vi "SENS_CORR_COLL_GUID_CONN_CAT_ARY.vi"(0 "VNA":refnum<visa-resource-name>, 5 "error in":errorcluster, 7 "Channel":i32) -> (14 "VNA Out":refnum<visa-resource-name>, 16 "ConAry":string[](array[string]), 19 "error out":errorcluster)   [LabVIEW 2018, in "PNA-X.lvlib"]
uses:
  PNA-X.lvlib
panel:
  out "read buffer":string
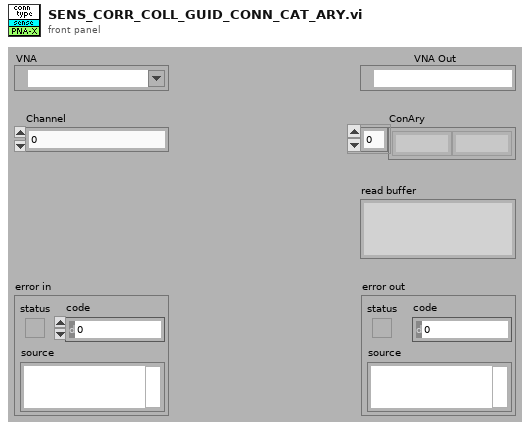
[diagram p1: front panel]
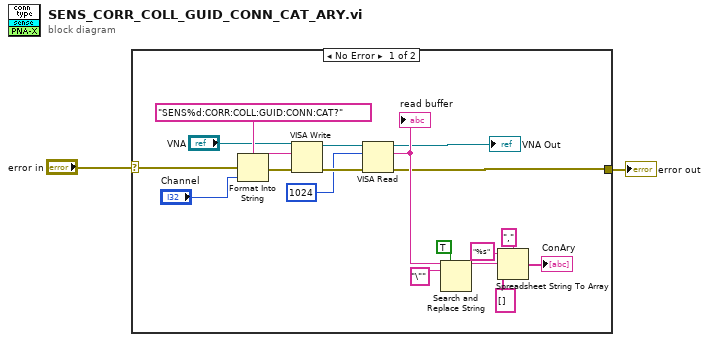
[diagram p0: block diagram]
diagram:
  n1 = case shown="No Error" "error in" {
    selector: "error in" -> [w6 w22]
    tunnel: [w3 w22] -> w1
    frame No Error {
      n2 = Format Into String(format string="SENS%d:CORR:COLL:GUID:CONN:CAT?", error in=w6, "Channel") -> (resulting string=w18:string, error out=w19:errorcluster)  [unwired: 1 in]
      n3 = VISA Write(VISA resource name="VNA", write buffer=w18, error in (no error)=w19) -> (VISA resource name out=w16:refnum<visa-resource-name>, error out=w17:errorcluster)  [unwired: 1 out]
      n4 = VISA Read(VISA resource name=w16, byte count=u32 1024, error in (no error)=w17) -> (VISA resource name out=→"VNA Out":refnum<visa-resource-name>, read buffer=w14:string, error out=w3:errorcluster)  [unwired: 1 out]
      "read buffer" <- w14
      n5 = Search and Replace String(replace all?=TRUE ("replace all? (F)"), input string=w14, search string="\"") -> (result string=w11:string)  [unwired: 5 in, 3 out]
      n6 = Spreadsheet String To Array(delimiter (Tab)=",", format string="%s", spreadsheet string=w11, array type (2D Dbl)=string[] []) -> (array=→"ConAry":string[])
    }
    frame Error {
    }
  }
  "error out" <- w1
